vi "set_config_cluster.vi"(8 "error in (no error)":errorcluster, 10 "config cluster variant":variant, 11 "SignalWriterDL090202DAQmx in":refnum<class "SignalWriterDL090202DAQmx.lvclass">) -> (0 "error out":errorcluster, 3 "SignalWriterDL090202DAQmx out":refnum<class "SignalWriterDL090202DAQmx.lvclass">)   [LabVIEW 2010, in "SignalWriterDL090202DAQmx.lvclass"]
uses:
  SignalWriterDL090202DAQmx.lvclass
  SignalWriterDL090202DAQmx.lvclass/SignalWriterDL090202DAQmx.ctl
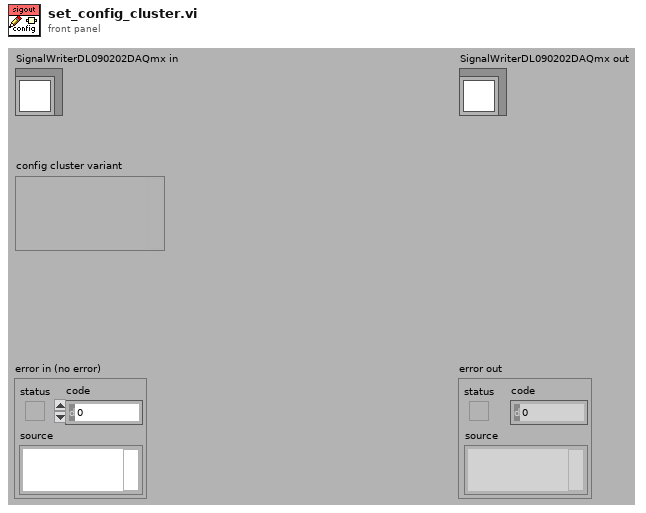
[diagram p1: front panel]
types:
  T1 = typedef "SignalWriterDL090202DAQmx.lvclass/config_data_cluster.ctl" = cluster{"physical channel":string, "timing source":string, "lag ":dbl[unit], "output type":string, "maximum output value":dbl, "minimum output value":dbl, "trigger line":string, "edge":T2, "counter":string}
  T2 = typedef "SignalWriterDL090202DAQmx.lvclass/trigger_edge_enum.ctl" = enum16{"rising", "falling"}
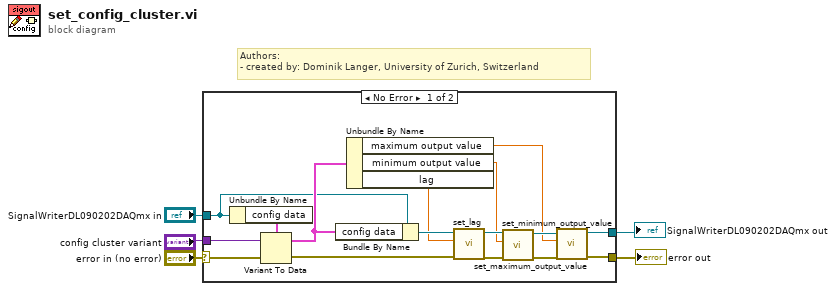
[diagram p0: block diagram]
diagram:
  # "Authors: \n- created by: Dominik Langer, University of Zurich, Switzerland"
  n1 = case shown="No Error" "error in (no error)" {
    selector: "error in (no error)" -> [w13 w23]
    tunnel: [w16 w23] -> w4
    tunnel: [w15 w22] -> w5
    tunnel: "SignalWriterDL090202DAQmx in" -> [w9 w22]
    tunnel: "config cluster variant" -> [w14 _]
    frame No Error {
      n2 = Unbundle By Name(w9) -> ("config data"=w12:T1)
      n3 = Variant To Data(error in=w13, Variant=w14, type=w12) -> (error out=w21:errorcluster, data=w11:T1)
      n4 = Bundle By Name(cluster=w9, "config data"=w11) -> (w10:refnum<class "SignalWriterDL090202DAQmx.lvclass">)
      n5 = Unbundle By Name(w11) -> ("maximum output value"=w6:dbl, "minimum output value"=w7:dbl, "lag"=w8:dbl[unit])
      n6 = call-dynamic "set_lag.vi"("error in (no error)"=w21, "lag"=w8, "DAQmxWriteSignals.lvclass in"=w10) -> ("error out"=w20:errorcluster, "DAQmxWriteSignals.lvclass out"=w17:refnum<class "SignalWriterDL090202DAQmx.lvclass">)  [unwired: 7 out]
      n7 = call-dynamic "set_minimum_output_value.vi"("error in (no error)"=w20, "minimum output value"=w7, "DAQmxWriteSignals.lvclass in"=w17) -> ("error out"=w19:errorcluster, "DAQmxWriteSignals.lvclass out"=w18:refnum<class "SignalWriterDL090202DAQmx.lvclass">)  [unwired: 7 out]
      n8 = call-dynamic "set_maximum_output_value.vi"("error in (no error)"=w19, "maximum output value"=w6, "DAQmxWriteSignals.lvclass in"=w18) -> ("error out"=w16:errorcluster, "DAQmxWriteSignals.lvclass out"=w15:refnum<class "SignalWriterDL090202DAQmx.lvclass">)  [unwired: 7 out]
    }
    frame Error {
    }
  }
  "error out" <- w4
  "SignalWriterDL090202DAQmx out" <- w5
